vi "Close Connection.vi"(4 "error in (no error)":errorcluster, 7 "Connection Refnum":T1) -> (0 "error out":errorcluster)   [LabVIEW 2011]
doc: "Se déconnecte de la base spécifiée en libérant les liens crées"
uses:
  Win32/ODBC/SQL Controls/Connection Refnum.ctl
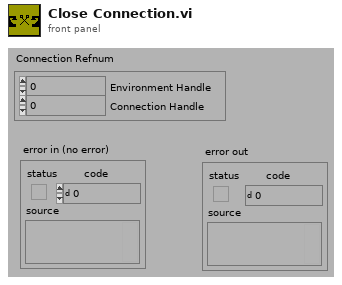
[diagram p1: front panel]
types:
  T1 = typedef "Connection Refnum.ctl" = cluster{"Environment Handle":i32, "Connection Handle":i32}
  T2 = enum16{"NOPE", "SQL_HANDLE_ENV", "SQL_HANDLE_DBC", "SQL_HANDLE_STMT", "SQL_HANDLE_DESC"}
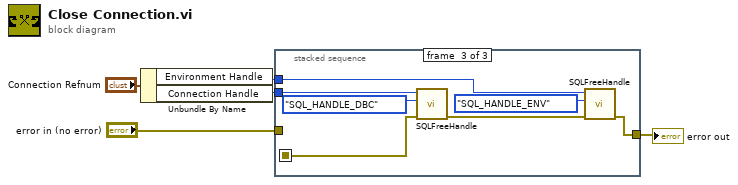
[diagram p0: block diagram]
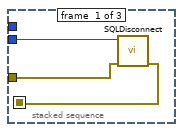
[diagram p2: hidden frame]
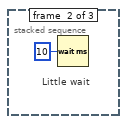
[diagram p3: hidden frame]
diagram:
  n1 = Unbundle By Name("Connection Refnum") -> ("Environment Handle"=w4:i32, "Connection Handle"=w3:i32)
  n2 = stacked-sequence {
    seq-local: [w6 _ _] -> [_ _ w15]
    tunnel: w3 -> [w8 _ w16]
    tunnel: w4 -> [_ _ w13]
    tunnel: "error in (no error)" -> [w7 _ _]
    tunnel: [_ _ w10] -> w1
    frame #0 {
      n3 = call "SQLDisconnect.vi"("error in (no error)"=w7, "InputHandle"=w8) -> ("error out"=w6:errorcluster)  [unwired: 1 in, 4 out]
    }
    frame #1 {
      # "Little wait"
      n4 = Wait (ms)(milliseconds to wait=u32 10) -> ()  [unwired: 1 out]
    }
    frame #2 {
      n5 = call "SQLFreeHandle.vi"("error in (no error)"=w15, "HandleType"=T2."SQL_HANDLE_DBC", "InputHandle"=w16) -> ("error out"=w12:errorcluster)  [unwired: 2 in, 2 out]
      n6 = call "SQLFreeHandle.vi"("error in (no error)"=w12, "HandleType"=T2."SQL_HANDLE_ENV", "InputHandle"=w13) -> ("error out"=w10:errorcluster)  [unwired: 4 out]
    }
  }
  "error out" <- w1
